vi "String.String to 2D.vi"(7 "DelimCol":string=";", 10 "DelimRow":string="|", 11 "String":string) -> (3 "Array":string[][](array[string]))   [LabVIEW 2019]
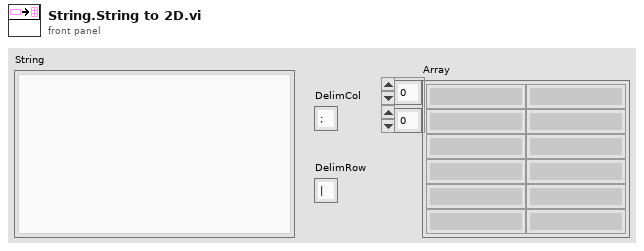
[diagram p1: front panel]
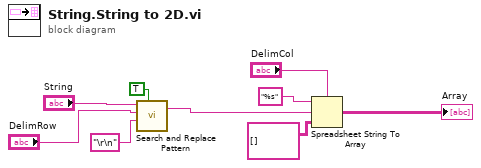
[diagram p0: block diagram]
diagram:
  n1 = call <vilib>:"Search and Replace Pattern.vi"("string"="String", "regular expression (\"\")"="DelimRow", "replace string (\"\")"="\r\n" ("regular expression (\"\")"), "replace all? (F)"=TRUE) -> ("result string"=w6:string)  [unwired: 1 in, 1 out]
  n2 = Spreadsheet String To Array(delimiter (Tab)="DelimCol", format string="%s", spreadsheet string=w6, array type (2D Dbl)=string[][] [] ("Array")) -> (array=→"Array":string[][])
